vi "Init IO Ports.vi"(11 "VISA Refnum in":refnum<visa-resource-name>="COM1") -> (3 "IO Port Cluster":T8)   [LabVIEW 2013]
uses:
  <vilib>/myRIO/Instrument Drivers/Onboard IO/PWM/typedefs/PWM Reference.ctl
  <vilib>/myRIO/Common/Instrument Driver Framework/Utilities/typedefs/myRIO Generic Hardware Reference.ctl
  <vilib>/myRIO/Common/Instrument Driver Framework/Utilities/typedefs/Hardware Version Enum.ctl
  <vilib>/myRIO/Common/Instrument Driver Framework/Utilities/typedefs/myRIO v1.0 Reference.ctl
  <vilib>/myRIO/Common/Instrument Driver Framework/Utilities/typedefs/Generic FPGA Reference.ctl
  <vilib>/myRIO/Common/Instrument Driver Framework/myRIO v1.0/PWM/typedefs/PWM Channels Enum.ctl
  <vilib>/myRIO/Instrument Drivers/Onboard IO/PWM/typedefs/PWM Configuration.ctl
  <vilib>/myRIO/Common/Instrument Driver Framework/myRIO v1.0/PWM/vis/myRIO v1.1 Open PWM.vi
  <vilib>/myRIO/Common/Instrument Driver Framework/Utilities/vis/Validate Channels.vi
  <vilib>/myRIO/Common/Instrument Driver Framework/myRIO v1.0/PWM/vis/myRIO v1.0 Reserve PWM.vi
  <vilib>/myRIO/Common/Instrument Driver Framework/myRIO v1.0/PWM/vis/myRIO v1.0 Build MUX Configuration PWM.vi
  <vilib>/myRIO/Common/Instrument Driver Framework/myRIO v1.0/Resource Manager/vis/myRIO v1.0 Reserve Channel List.vi
  <vilib>/myRIO/Common/Instrument Driver Framework/myRIO v1.0/Resource Manager/vis/myRIO v1.0 Create Configuration List.vi
  <vilib>/myRIO/Common/Instrument Driver Framework/myRIO v1.0/Resource Manager/vis/myRIO v1.0 Reserve Channel.vi
  <vilib>/myRIO/Common/Instrument Driver Framework/myRIO v1.0/Resource Manager/vis/myRIO v1.0 Unreserve Channel.vi
  <vilib>/myRIO/Common/Instrument Driver Framework/myRIO v1.0/Resource Manager/vis/myRIO v1.0 Build Mutex Name.vi
  <vilib>/Instr/_visa.llb/VISA Configure Serial Port (Instr).vi
  <vilib>/myRIO/Common/Instrument Driver Framework/myRIO v1.0/myRIO v1.1 Open.vi
  <vilib>/Utility/VariantDataType/GetNumericInfo.vi
  <vilib>/Utility/error.llb/Error Cluster From Error Code.vi
  <vilib>/myRIO/Common/Instrument Driver Framework/Utilities/vis/IO Manager.vi
  <vilib>/myRIO/Common/Instrument Driver Framework/Utilities/vis/Configuration Manager.vi
  <vilib>/myRIO/Common/Instrument Driver Framework/myRIO v1.0/Resource Manager/vis/myRIO v1.0 Configure IO.vi
  <vilib>/myRIO/Common/Instrument Driver Framework/myRIO v1.0/myRIO v1.0 Close.vi
  <vilib>/myRIO/Instrument Drivers/Onboard IO/PWM/PWM.lvlib
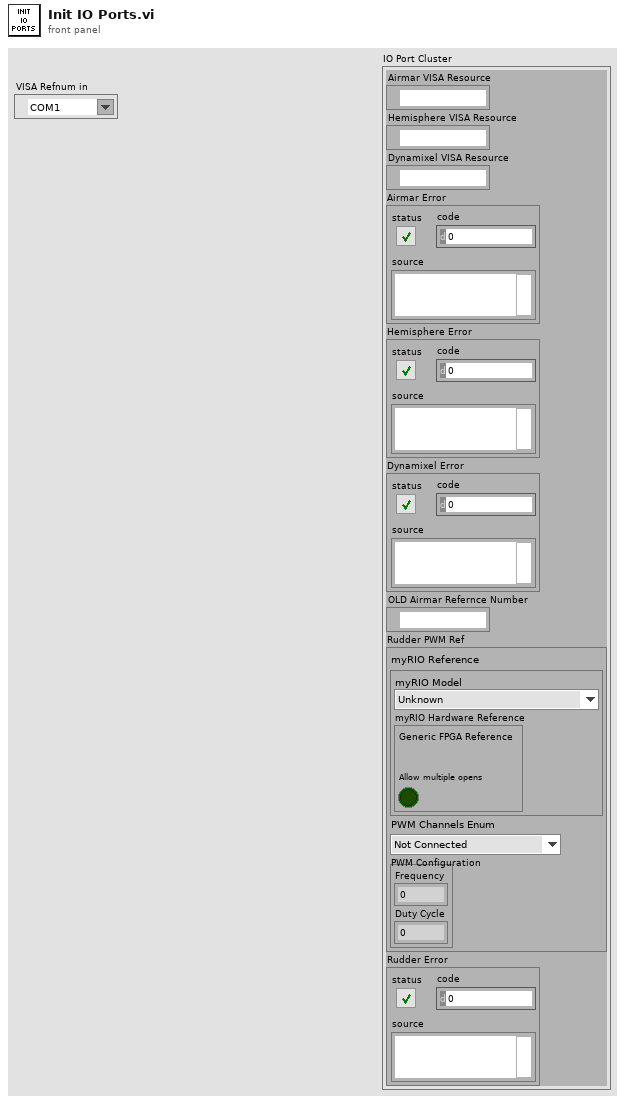
[diagram p1: front panel]
types:
  T1 = typedef "PWM.lvlib/PWM Reference.ctl" = cluster{"myRIO Reference":T2, "PWM Channels Enum":T6, "PWM Configuration":T7}
  T2 = typedef "myRIO Generic Hardware Reference.ctl" = cluster{"myRIO Model":T3, "myRIO Hardware Reference":T4}
  T3 = typedef "Hardware Version Enum.ctl" = enum16{"Unknown", "myRIO-1900", "myRIO-1950"}
  T4 = typedef "myRIO v1.0 Reference.ctl" = cluster{"Generic FPGA Reference":T5, "Allow multiple opens":bool}
  T5 = typedef "Generic FPGA Reference.ctl" = refnum<k20>
  T6 = typedef "PWM Channels Enum.ctl" = enum16{"Not Connected", "C/PWM0", "C/PWM1", "A/PWM0", "A/PWM1", "A/PWM2", "B/PWM0", "B/PWM1", "B/PWM2"}
  T7 = typedef "PWM.lvlib/PWM Configuration.ctl" = cluster{"Frequency":dbl, "Duty Cycle":dbl}
  T8 = cluster{"Airmar VISA Resource":refnum<visa-resource-name>, "Hemisphere VISA Resource":refnum<visa-resource-name>, "Dynamixel VISA Resource":refnum<visa-resource-name>, "Airmar Error":errorcluster, "Hemisphere Error":errorcluster, "Dynamixel Error":errorcluster, "OLD Airmar Refernce Number":refnum<visa-resource-name>, "Rudder PWM Ref":T1, "Rudder Error":errorcluster}
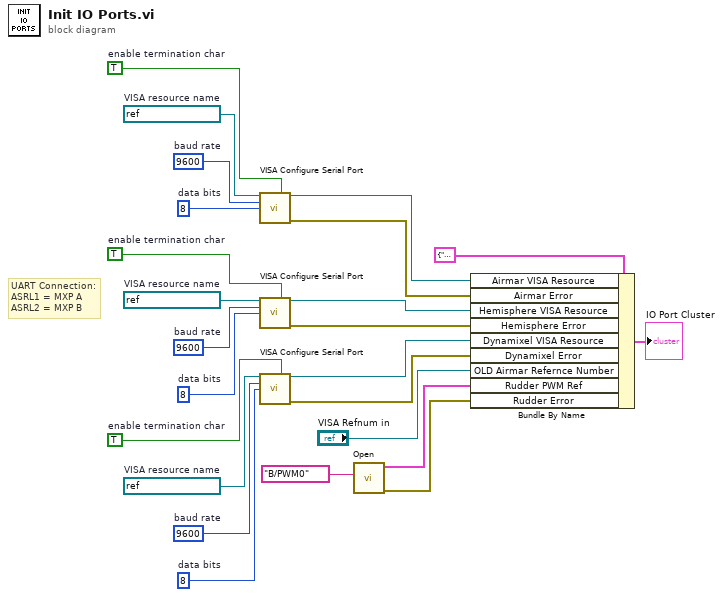
[diagram p0: block diagram]
diagram:
  w21 = TRUE  # enable termination char
  w22 = u16 8  # data bits
  w23 = u32 9600  # baud rate
  w24 = refnum<visa-resource-name> "ASRL1::INSTR"  # VISA resource name
  w20 = TRUE  # enable termination char
  w19 = u16 8  # data bits
  w18 = u32 9600  # baud rate
  w17 = refnum<visa-resource-name> "ASRL1::INSTR"  # VISA resource name
  w15 = TRUE  # enable termination char
  w14 = u16 8  # data bits
  w13 = u32 9600  # baud rate
  w12 = refnum<visa-resource-name> "ASRL1::INSTR"  # VISA resource name
  # "UART Connection:\nASRL1 = MXP A \nASRL2 = MXP B"
  n1 = call-poly "VISA Configure Serial Port"("VISA resource name"=w17, "Enable Termination\nChar (T)"=w20, "baud rate (9600)"=w18, "data bits (8)"=w19) -> ("VISA resource name out"=w10:refnum<visa-resource-name>, "error out"=w9:errorcluster)  [unwired: 10 in]
  n2 = call-poly "VISA Configure Serial Port"("VISA resource name"=w24, "Enable Termination\nChar (T)"=w21, "baud rate (9600)"=w23, "data bits (8)"=w22) -> ("VISA resource name out"=w8:refnum<visa-resource-name>, "error out"=w7:errorcluster)  [unwired: 10 in]
  n3 = call-poly "VISA Configure Serial Port"("VISA resource name"=w12, "Enable Termination\nChar (T)"=w15, "baud rate (9600)"=w13, "data bits (8)"=w14) -> ("VISA resource name out"=w6:refnum<visa-resource-name>, "error out"=w5:errorcluster)  [unwired: 10 in]
  n4 = call <vilib>:"Open.vi"("Channel Name"=tag "B/PWM0" ("PWM channel")) -> ("error out"=w2:errorcluster, "PWM Ref Out"=w3:T1)  [unwired: 9 in]
  n5 = Bundle By Name(cluster=T8 {"Airmar VISA Resource"="", "Hemisphere VISA Resource"="", "Dynamixel VISA Resource"="", "Airmar Error"={"status"=FALSE, "code"=0, "source"=""}, "Hemisphere Error"={"status"=FALSE, "code"=0, "source"=""}, "Dynamixel Error"={"status"=FALSE, "code"=0, "source"=""}, "OLD Airmar Refernce Number"="COM1", "Rudder PWM Ref"={"myRIO Reference"={"myRIO Model"=enum."Unknown", "myRIO Hardware Reference"={"Generic FPGA Reference"=refnum, "Allow multiple opens"=FALSE}}, "PWM Channels Enum"=enum."Not Connected", "PWM Configuration"={"Frequency"=0.0, "Duty Cycle"=0.0}}, "Rudder Error"={"status"=FALSE, "code"=0, "source"=""}}, "Airmar VISA Resource"=w10, "Airmar Error"=w9, "Hemisphere VISA Resource"=w8, "Hemisphere Error"=w7, "Dynamixel VISA Resource"=w6, "Dynamixel Error"=w5, "OLD Airmar Refernce Number"="VISA Refnum in", "Rudder PWM Ref"=w3, "Rudder Error"=w2) -> (→"IO Port Cluster":T8)
